vi "toggle_brakes.vi"(1 "set_brakes":bool) -> (0 "current_brake_state":bool)   [LabVIEW 2018]
uses:
  <vilib>/rvi/eio/common/nirviEmuTemplateMethod_errors.vi
  <vilib>/eio/EIONode/EIONode.xnode
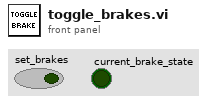
[diagram p1: front panel]
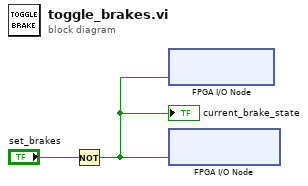
[diagram p0: block diagram]
diagram:
  n1 = Not(x="set_brakes") -> (.not. x?=w1:bool)
  "current_brake_state" <- w1
  n2 = xnode "FPGA I/O Node"("Mod2/DIO9"=w1) -> ()  [unwired: 1 in, 1 out]
  n3 = xnode "FPGA I/O Node"("Mod2/DIO10"=w1) -> ()  [unwired: 1 in, 1 out]
